vi "get_Power.vi"(6 "reset":bool, 8 "error in":errorcluster, 10 "Simulation mode":bool, 11 "Average Time (sec)":dbl) -> (0 "error out":errorcluster, 3 "Power":dbl)   [LabVIEW 2021]
doc: "Random Laser Project v2.0\nAndré Romero - 2024\nandretec@ifsc.usp.br"
uses:
  Global_v20.vi
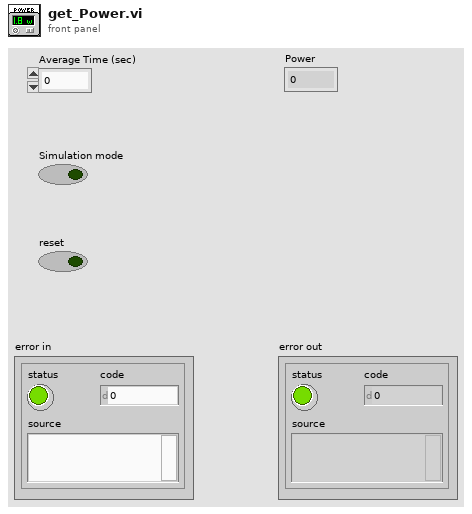
[diagram p1: front panel]
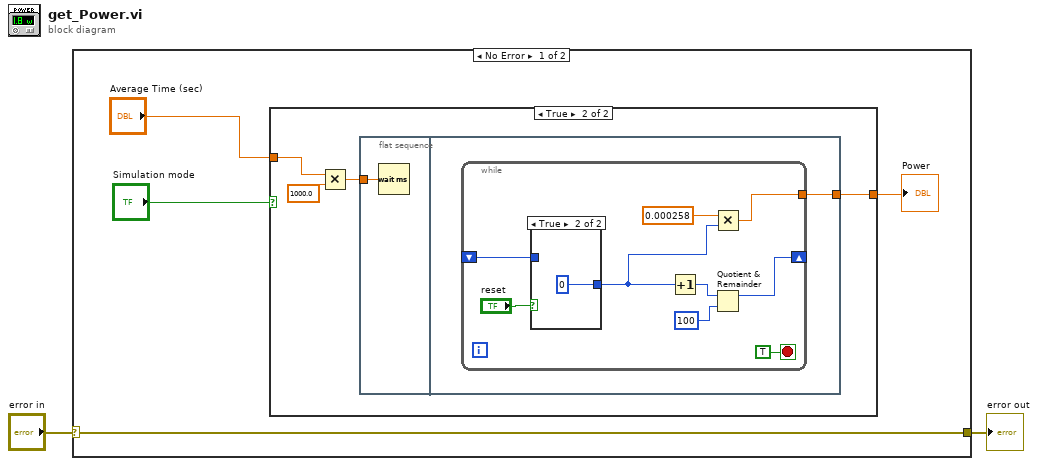
[diagram p0: block diagram]
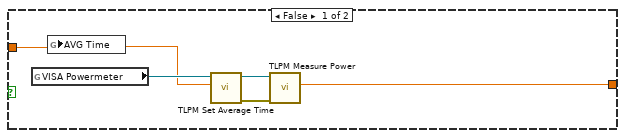
[diagram p2: hidden frame]
diagram:
  n1 = case shown="No Error" "error in" {
    selector: "error in" -> [w3 w29]
    tunnel: [w3 w29] -> w1
    frame No Error {
      n2 = case shown="True" "Simulation mode" {
        tunnel: [w8 w12] -> w5
        tunnel: "Average Time (sec)" -> [w7 w14]
        frame False {
          n3 = global read "Global_v20.vi" "VISA Powermeter"() -> (w11:refnum<visa-resource-name>)
          n4 = global write "Global_v20.vi" "AVG Time"(w7) -> ()
          n5 = call <instrlib>:"TLPM Set Average Time.vi"("Average Time (0.0)"=w7, "instrument handle"=w11) -> ("error out"=w9:errorcluster, "instrument handle out"=w10:refnum<visa-resource-name>)  [unwired: 8 in]
          n6 = call <instrlib>:"TLPM Measure Power.vi"("error in (no error)"=w9, "instrument handle"=w10) -> ("Power"=w8:dbl)  [unwired: 7 in, 2 out]
        }
        frame True {
          n7 = Multiply(x=w14, y=1000.0) -> (x*y=w13:dbl)
          n8 = flat-sequence {
            tunnel: w13 -> [w16]
            tunnel: [w17] -> w12
            frame #0 {
              n9 = Wait (ms)(milliseconds to wait=w16) -> ()  [unwired: 1 out]
            }
            frame #1 {
              n10 = while {
                shift-right: [w22] -> _
                shift-left: _ -> [w18]
                tunnel: [w21] -> w17
                stop <- TRUE stop-if-true
                n11 = case shown="True" "reset" {
                  tunnel: [w27 0] -> w19
                  tunnel: w18 -> [w27 _]
                  frame False {
                  }
                  frame True {
                  }
                }
                n12 = Increment(x=w19) -> (x+1=w24:i32)
                n13 = Multiply(x=0.000258, y=w19) -> (x*y=w21:dbl)
                n14 = Quotient & Remainder(x=w24, y=100) -> (x-y*floor(x/y)=w22:i32)  [unwired: 1 out]
              }
            }
          }
        }
      }
      "Power" <- w5
    }
    frame Error {
    }
  }
  "error out" <- w1
